vi "CheckSecPlatMotor.vi"(8 "错误输入（无错误）":errorcluster, 11 "Bool引用":refnum<vi>) -> (0 "错误输出":errorcluster)   [LabVIEW 2011]
uses:
  API/API DYM.lvlib
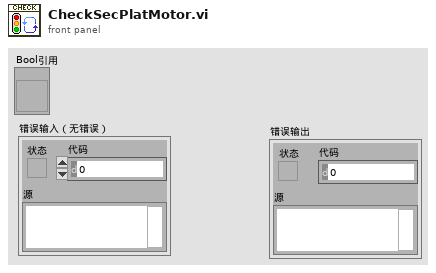
[diagram p1: front panel]
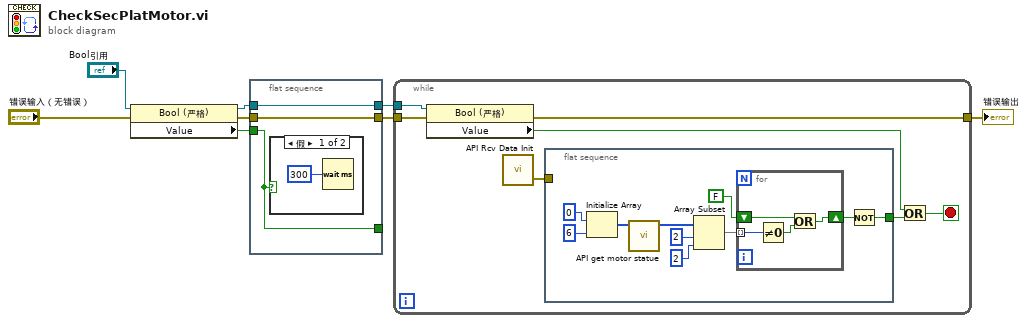
[diagram p0: block diagram]
diagram:
  n1 = property on="属性节点" class="Bool (严格)"(reference="Bool引用", error in="错误输入（无错误）") -> (reference out=w6:refnum<vi>, error out=w5:errorcluster, "Value"=w4:bool)
  n2 = flat-sequence {
    tunnel: w6 -> [w9]
    tunnel: [w11] -> w3
    tunnel: w5 -> [w11]
    tunnel: w4 -> [w10]
    tunnel: [w10] -> _
    tunnel: [w9] -> w2
    frame #0 {
      n3 = case shown="假" w10 {
        frame False {
          n4 = Wait (ms)(milliseconds to wait=u32 300 ("等待时间（毫秒）")) -> ()  [unwired: 1 out]
        }
        frame True {
        }
      }
    }
  }
  n5 = while {
    tunnel: w3 -> [w18]
    tunnel: w2 -> [w19]
    tunnel: [w17] -> w1
    stop <- w14 stop-if-true
    n6 = property on="属性节点" class="Bool (严格)"(reference=w19, error in=w18) -> (error out=w17:errorcluster, "Value"=w15:bool)  [unwired: 1 out]
    n7 = call "API Rcv Data Init.vi"() -> ("错误输出"=w13:errorcluster)  [unwired: 2 in, 1 out]
    n8 = flat-sequence {
      tunnel: [w20] -> w16
      tunnel: w13 -> [_]
      frame #0 {
        n9 = Initialize Array(0, 6 ("维数大小")) -> (w27:i32[])
        n10 = call "API get motor statue.vi"("motor statue array input"=w27) -> ("motor statue array output"=w26:i32[])  [unwired: 9 in, 1 out]
        n11 = Array Subset(array=w26, index=2 ("索引"), length=2 ("长度")) -> (w23:i32[])
        n12 = for {
          shift-right: [w31] -> w21
          shift-left: FALSE -> [w32]
          tunnel: w23 -> [w30] mode=indexing
          n13 = Not Equal To 0?(x=w30) -> (x != 0?=w33:bool)
          n14 = Or(x=w32, y=w33) -> (x .or. y?=w31:bool)
        }
        n15 = Not(x=w21) -> (.not. x?=w20:bool)
      }
    }
    n16 = Or(x=w15, y=w16) -> (x .or. y?=w14:bool)
  }
  "错误输出" <- w1
